vi "XYZtoStrings.vi"(9 "Pøenos (dB)":dbl[](array[numeric]), 10 "Amplituda (V)":dbl[](array[numeric]), 11 "Frekvence (Hz)":dbl[](array[numeric])) -> (3 "concatenated string":string)   [LabVIEW 2021]
panel:
  out "appended array":dbl[][](array[numeric])
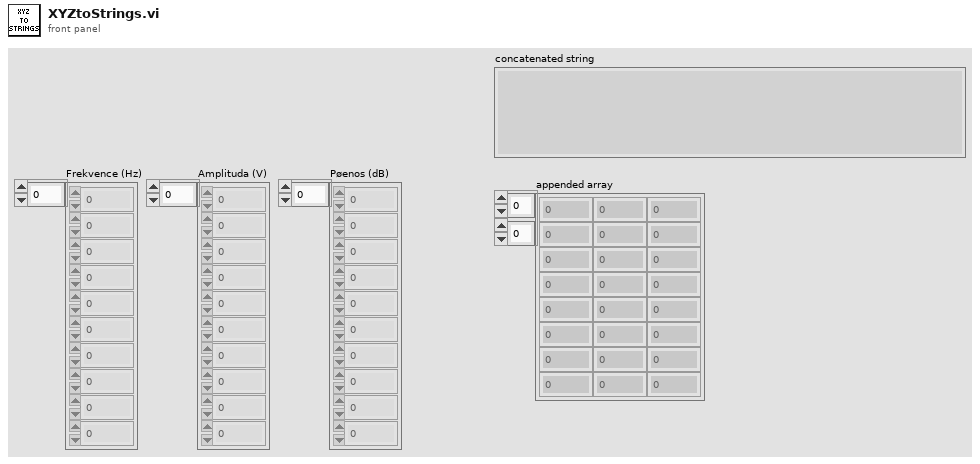
[diagram p1: front panel]
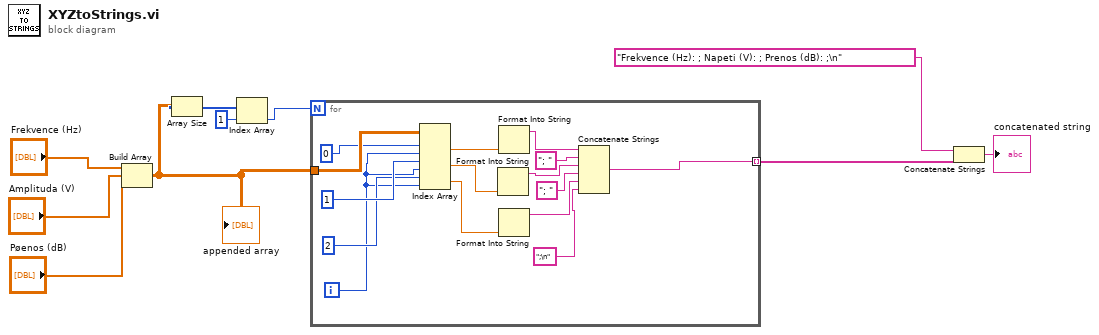
[diagram p0: block diagram]
diagram:
  n1 = Build Array("Frekvence (Hz)", "Amplituda (V)", "Pøenos (dB)") -> (w5:dbl[][])
  "appended array" <- w5
  n2 = Array Size(array=w5) -> (size(s)=w8:i32[])
  n3 = Index Array(array=w8, index=1) -> (element=w6:i32)
  n4 = for {
    N: w6 -> [_]
    tunnel: w5 -> [w25]
    tunnel: [w19] -> w4 mode=indexing
    i -> [w14]
    n5 = Index Array(array=w25, index (row) #1=0 ("disabled index (col)"), index (col) #1=w14, index (row) #2=1 ("disabled index (col)"), index (col) #2=w14, index (row) #3=2 ("index (row)"), index (col) #3=w14) -> (element #1=w24:dbl, element #2=w23:dbl, element #3=w13:dbl)
    n6 = Format Into String(w23) -> (resulting string=w20:string)  [unwired: 3 in, 1 out]
    n7 = Format Into String(w24) -> (resulting string=w22:string)  [unwired: 3 in, 1 out]
    n8 = Format Into String(w13) -> (resulting string=w12:string)  [unwired: 3 in, 1 out]
    n9 = Concatenate Strings(w22, "; " ("string"), w20, "; " ("string"), w12, ";\n" ("string")) -> (w19:string)
  }
  n10 = Concatenate Strings("Frekvence (Hz): ; Napeti (V): ; Prenos (dB): ;\n" ("string"), w4) -> (→"concatenated string":string)
